vi "Timeout Selector.vi"(6 "Remaining States":string, 7 "Timeout Expected":i32) -> (3 "Timeout":i32)   [LabVIEW 2014, in "JKI-State-Machine-Plus.lvlib"]
uses:
  JKI-State-Machine-Plus.lvlib
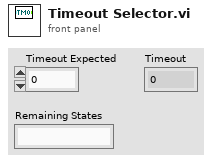
[diagram p1: front panel]
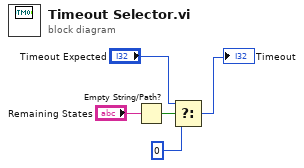
[diagram p0: block diagram]
diagram:
  n1 = Empty String/Path?(string/path="Remaining States") -> (empty?=w2:bool)
  n2 = Select(t="Timeout Expected", s=w2, f=0) -> (s? t:f=→"Timeout":i32)
